vi "Manual-Automatic Control with Engineering Units.vi"() -> ()   [LabVIEW 2023]
doc: "This example demonstrates how to simulate a simple control loop with a general plant model with real engineering units. This example uses the PID Advanced VI to switch between manual and automatic control."
uses:
  <vilib>/addons/control/pid/pid.llb/PID Structure.ctl
  <vilib>/addons/control/pid/pid.llb/PID Time Unit.ctl
  <vilib>/addons/control/pid/pid.llb/PID Gain Unit.ctl
  <vilib>/addons/control/pid/pid.llb/PID Structure Conversion (DBL).vi
  <vilib>/addons/control/pid/pid.llb/PID EGU to Percentage (DBL).vi
  <vilib>/addons/control/pid/pid.llb/PID Advanced (DBL).vi
  <vilib>/addons/control/pid/pid.llb/PID Percentage to EGU (DBL).vi
  <vilib>/addons/control/pid/NI_PID_pid.lvlib
panel:
  in  "PID Structure":T1 items=["Academic (Standard)", "Parallel", "Series"]
  in  "Proportional Unit":T2=1 items=["Gain (Kc)", "Band (PB)"]
  in  "Derivative Unit":T3 items=["min", "s"]
  in  "Integral Unit":T3 items=["min", "s"]
  in  "Derivative":dbl format="%#.3g"
  in  "Integral":dbl=0.05 format="%#.3g"
  in  "Proportional":dbl=5.0 format="%.3f"
  in  "Input Unit":enum16{"%", "EGU"}(ring)
  in  "Max In":dbl=1000.0 format="%#.3f"
  in  "Min In":dbl format="%#.3p"
  in  "Output Unit":enum16{"%", "EGU"}(ring)=enum."EGU"
  in  "Max Out":dbl=0.02 format="%#.3p"
  in  "Min Out":dbl=0.004 format="%#.3p"
  out "Process Variable and Setpoint":cluster{"initial PV":dbl, "SP1:":dbl}(graph)={"initial PV"=59.90039568060552, "SP1:"=63.81578947368421}
  in  "auto? (T)":bool=TRUE
  in  "SP:":dbl(slide)=63.81578947368421 scale=0.0..100.0
  in  "MV:":dbl(slide)=81.2966931242091 scale=-100.0..100.0 scale format="%#.3p"
  out "PV:":dbl(slide)=59.90039568060552 scale=0.0..100.0
  in  "Stop":bool
  out "Controller Output":dbl(graph)=0.018503735449936727
  # "Overview: This example demonstrates how to simulate a control loop with a general plant model with real engineering units. Note that the PID algorithm is non-dimensional and, if you do not need to switch between percentage and Engineering units, you just use engineering units on the gains and limits.\nInstructions:\n1. Run the VI and observe the Process Variable (PV) following the Setpoint (SP).\n2. Change the Input Unit and Output Unit values to see the charts change their limits.\n3. Click Stop to stop the VI."
  # "Automatic"
  # "Manual"
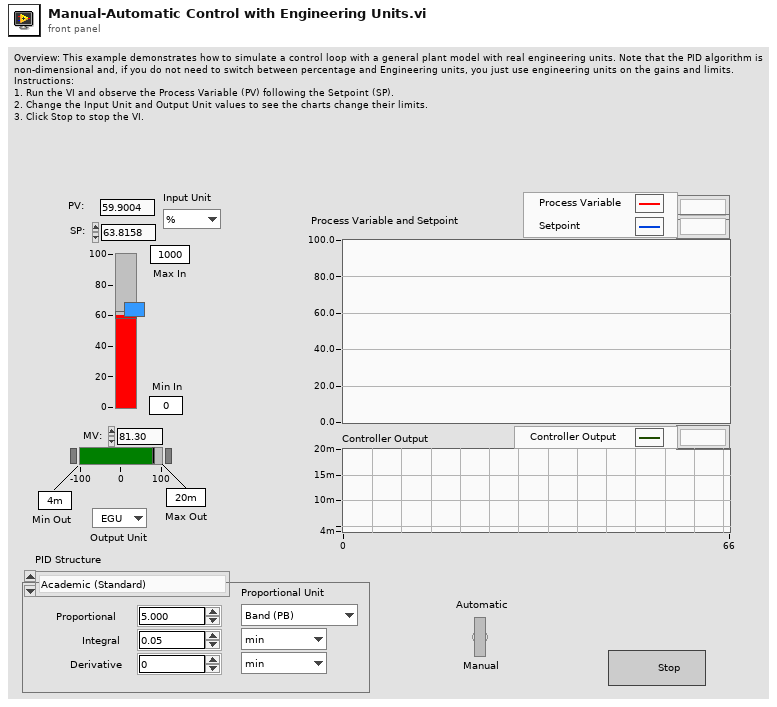
[diagram p1: front panel]
types:
  T1 = typedef "NI_PID_pid.lvlib/PID Structure.ctl" = u16
  T2 = typedef "NI_PID_pid.lvlib/PID Gain Unit.ctl" = u16
  T3 = typedef "NI_PID_pid.lvlib/PID Time Unit.ctl" = u16
  T4 = cluster{"static gain":dbl, "lag (min)":dbl, "dead cycles":i32, "load %":dbl, "deadband":dbl, "noise level %":dbl, "initial PV":dbl}
  T5 = cluster{"proportional gain (Kc)":dbl, "integral time (Ti, min)":dbl, "derivative time (Td, min)":dbl}
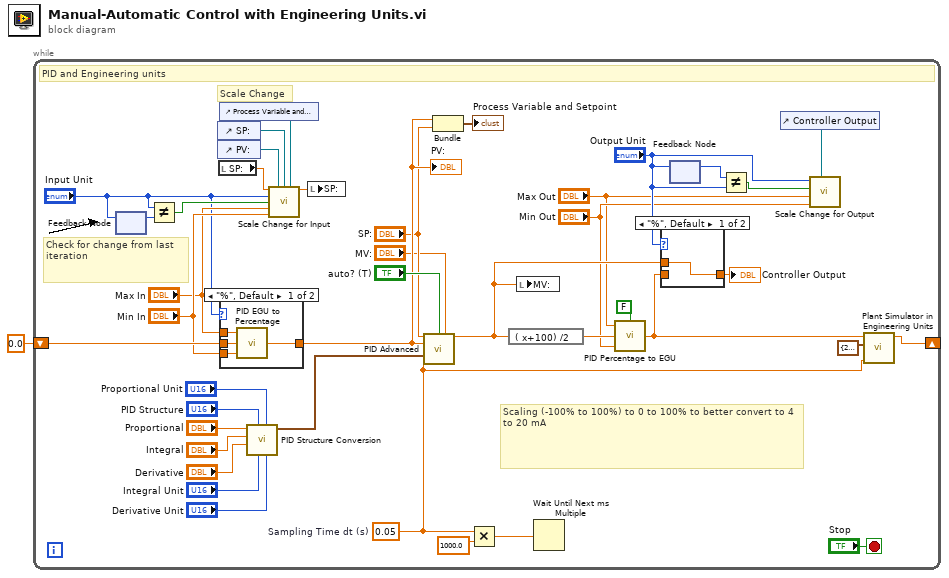
[diagram p0: block diagram]
diagram:
  n1 = while {
    shift-left: 0.0 ("Plant Output (EGU)") -> [w27]
    shift-right: [w37] -> _
    stop <- "Stop" stop-if-true
    w39 = 0.05  # Sampling Time dt (s)
    # "Check for change from last iteration"
    # "Scale Change"
    # "Scaling (-100% to 100%) to 0 to 100% to better convert to 4 to 20 mA"
    # "PID and Engineering units"
    n2 = feedback-in #1("Input Unit") -> ()
    n3 = feedback #1() -> (w13:enum16{"%", "EGU"})  [unwired: 1 out]
    n4 = Not Equal?(x="Input Unit", y=w13) -> (x != y?=w16:bool)
    n5 = control-ref of="SP:"() -> (w18:refnum<vi>)
    n6 = control-ref of="PV:"() -> (w19:refnum<vi>)
    n7 = local read "SP:"() -> (w4:dbl)
    n8 = control-ref of="Process Variable and Setpoint"() -> (w17:refnum<vi>)
    n9 = case shown="\"%\", Default" "Input Unit" {
      tunnel: w27 -> [w48 w49]
      tunnel: [w47 w49] -> w26
      tunnel: "Max In" -> [w46 _]
      tunnel: "Min In" -> [w45 _]
      frame "%", Default {
        n10 = call-poly <vilib>:"PID EGU to Percentage.vi"("minimum (EGU)"=w45, "input (EGU)"=w48, "maximum (EGU)"=w46) -> ("% span"=w47:dbl)
      }
      frame "EGU" {
      }
    }
    "PV:" <- w26
    n11 = call-poly <vilib>:"PID Structure Conversion.vi"("derivative unit"="Derivative Unit", "proportional unit"="Proportional Unit", "integral unit"="Integral Unit", "PID structure"="PID Structure", "derivative"="Derivative", "integral"="Integral", "proportional"="Proportional") -> ("PID gains"=w34:T5)  [unwired: 4 in]
    n12 = call "Scale Change for Input.vi"("SP:"=w4, "Slide Refnum"=w19, "Slide Refnum 2"=w18, "WFChart Refnum"=w17, "Input Unit"="Input Unit", "Change Scales"=w16, "Max In"="Max In", "Min In"="Min In") -> ("SP After Scale Change"=w15:dbl)  [unwired: 3 in, 4 out]
    n13 = local write "SP:"(w15) -> ()
    n14 = call-poly <vilib>:"PID Advanced.vi"("setpoint"="SP:", "auto? (T)"="auto? (T)", "manual control"="MV:", "process variable"=w26, "PID gains"=w34, "dt (s)"=w39) -> ("output"=w10:dbl)  [unwired: 7 in, 2 out]
    n15 = Bundle("Plant Output (EGU)"=w26, "SP:"="SP:") -> (→"Process Variable and Setpoint":cluster{"Plant Output (EGU)":dbl, "SP:":dbl})  [unwired: 1 out]
    n16 = Multiply(x=w39, y=1000.0) -> (x*y=w3:dbl)
    n17 = expression code="( x+100) /2"(w10) -> (w22:dbl)
    n18 = local write "MV:"(w10) -> ()
    n19 = Wait Until Next ms Multiple(millisecond multiple=w3) -> ()  [unwired: 1 out]
    n20 = call-poly <vilib>:"PID Percentage to EGU.vi"("coerce output to range? (T)"=FALSE, "minimum (EGU)"="Min Out", "% span"=w22, "maximum (EGU)"="Max Out") -> ("output (EGU)"=w11:dbl)
    n21 = case shown="\"%\", Default" "Output Unit" {
      tunnel: w10 -> [w43 _]
      tunnel: [w43 w44] -> w12
      tunnel: w11 -> [_ w44]
      frame "%", Default {
      }
      frame "EGU" {
      }
    }
    "Controller Output" <- w12
    n22 = feedback-in #2("Output Unit") -> ()
    n23 = feedback #2() -> (w21:enum16{"%", "EGU"})  [unwired: 1 out]
    n24 = Not Equal?(x=w21, y="Output Unit") -> (x != y?=w8:bool)
    n25 = control-ref of="Controller Output"() -> (w7:refnum<vi>)
    n26 = call "Scale Change for Output.vi"("WFChart Refnum"=w7, "Min Out"="Min Out", "Max Out"="Max Out", "Boolean"=w8, "Output Unit"="Output Unit") -> ()  [unwired: 5 in, 2 out]
    n27 = call "Plant Simulator in Engineering Units.vi"("Sampling Time dt (s)"=w39, "process parameters"=T4 {"static gain"=2.5, "lag (min)"=0.3, "dead cycles"=1, "load %"=40.0, "deadband"=2.0, "noise level %"=0.25, "initial PV"=0.0}, "Plnat Input (EGU)"=w11) -> ("Plant Output (EGU)"=w37:dbl)  [unwired: 2 in, 6 out]
  }
